vi "Write Paramaters.vi"(8 "error in (no error)":errorcluster, 9 "diastole":dbl, 10 "systole":dbl, 11 "Sawtooth in":refnum<class "Sawtooth.lvclass">) -> (0 "error out":errorcluster, 3 "Sawtooth out":refnum<class "Sawtooth.lvclass">)   [LabVIEW 2020, in "Sawtooth.lvclass"]
uses:
  Sawtooth.lvclass
  Sawtooth.lvclass/Sawtooth.ctl
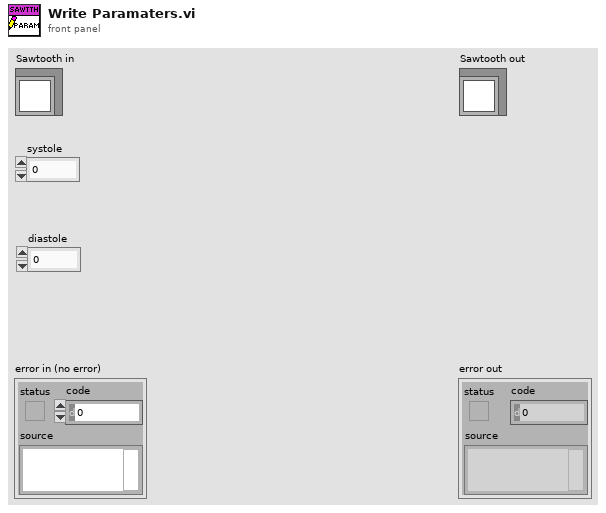
[diagram p1: front panel]
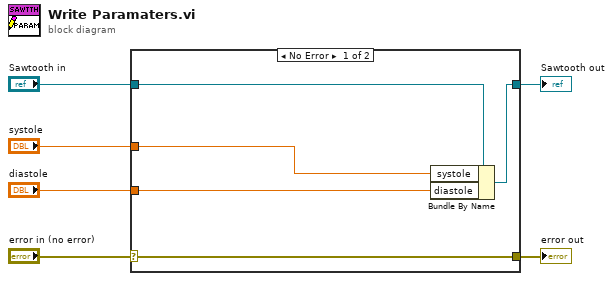
[diagram p0: block diagram]
diagram:
  n1 = case shown="No Error" "error in (no error)" {
    selector: "error in (no error)" -> [w11 w12]
    tunnel: [w11 w12] -> w5
    tunnel: [w9 w13] -> w3
    tunnel: "Sawtooth in" -> [w10 w13]
    tunnel: "systole" -> [w8 _]
    tunnel: "diastole" -> [w7 _]
    frame No Error {
      n2 = Bundle By Name(cluster=w10, "systole"=w8, "diastole"=w7) -> (w9:refnum<class "Sawtooth.lvclass">)
    }
    frame Error {
    }
  }
  "error out" <- w5
  "Sawtooth out" <- w3
